vi "SetFrontPanelTypeRingFromPluginINIFile.vi"(7 "Type Key":string="Type", 8 "ErrorArray In":errorcluster[](array[cluster]), 10 "INIFilePath":path, 11 "TypeRef In":refnum<vi>) -> (0 "ErrorArray Out":errorcluster[](array[cluster]), 3 "TypeRef Out":refnum<vi>)   [LabVIEW 2017, in "Framework.lvlib"]
uses:
  Framework.lvlib
  <vilib>/Utility/config.llb/Read Key (String).vi
  <vilib>/Utility/config.llb/NI_LVConfig.lvlib
  <userlib>/NIST/NISTErrorLib/NISTErrorLib.lvlib
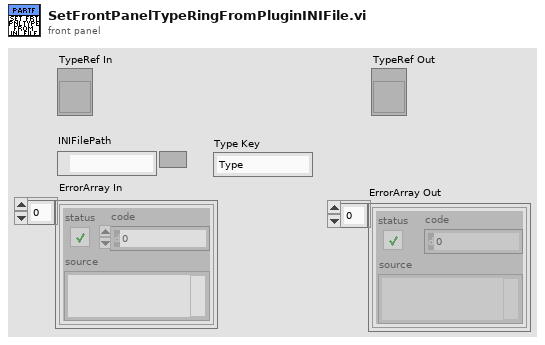
[diagram p1: front panel]
types:
  T1 = typedef "NI_LVConfig.lvlib/Config Data RefNum.ctl" = refnum<k1>
  T2 = typedef "LVStringsAndValuesArrayTypeDef_U16.ctl" = cluster{"String":string, "Value":u16}[]
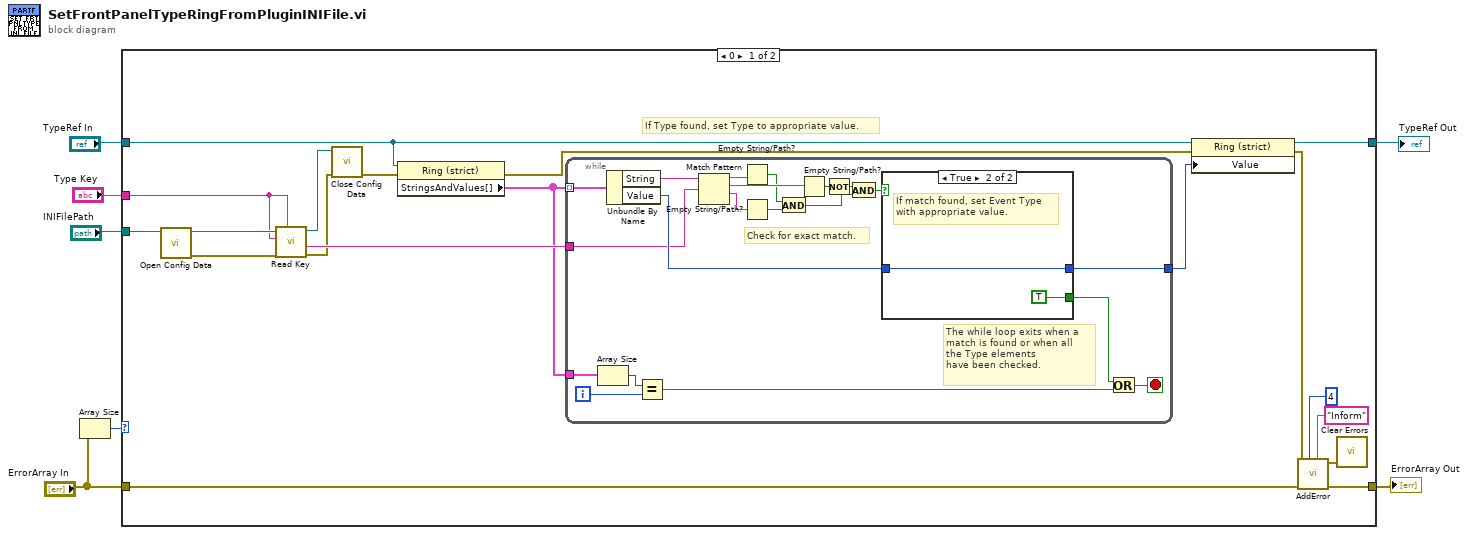
[diagram p0: block diagram]
diagram:
  n1 = Array Size(array="ErrorArray In") -> (size(s)=w6:i32)
  n2 = case shown="0" w6 {
    tunnel: [w21 w50] -> w7
    tunnel: "ErrorArray In" -> [w20 w50]
    tunnel: "INIFilePath" -> [w19 _]
    tunnel: "Type Key" -> [w11 _]
    tunnel: "TypeRef In" -> [w10 w49]
    tunnel: [w9 w49] -> w1
    frame 0 {
      # "If Type found, set Type to appropriate value."
      n3 = call <vilib>:"Open Config Data.vi"("configuration file path"=w19) -> ("error out"=w17:errorcluster, "refnum"=w18:T1)  [unwired: 8 in, 1 out]
      n4 = call-poly <vilib>:"Read Key.vi"("section"=w11, "error in (no error)"=w17, "key"=w11, "refnum"=w18) -> ("error out"=w25:errorcluster, "value"=w26:string, "refnum out"=w24:T1)  [unwired: 4 in, 1 out]
      n5 = call <vilib>:"Close Config Data.vi"("error in (no error)"=w25, "refnum"=w24) -> ("error out"=w23:errorcluster)  [unwired: 8 in, 1 out]
      n6 = property class="Ring (strict)"(reference=w10, error in=w23) -> (error out=w14:errorcluster, "StringsAndValues[]"=w22:T2)  [unwired: 1 out]
      n7 = while {
        tunnel: w22 -> [w46] mode=indexing
        tunnel: w26 -> [w35]
        tunnel: w22 -> [w30]
        tunnel: [w27] -> w13
        i -> [w31]
        stop <- w29 stop-if-true
        # "The while loop exits when a \nmatch is found or when all \nthe Type elements \nhave been checked."
        # "Check for exact match."
        n8 = Array Size(array=w30) -> (size(s)=w33:i32)
        n9 = Unbundle By Name(w46) -> ("String"=w45:string, "Value"=w43:u16)
        n10 = Equal?(x=w33, y=w31) -> (x = y?=w32:bool)
        n11 = Match Pattern(string=w45, regular expression=w35) -> (before substring=w40:string, match substring=w44:string, after substring=w39:string)  [unwired: 1 in, 1 out]
        n12 = Empty String/Path?(string/path=w40) -> (empty?=w37:bool)
        n13 = Empty String/Path?(string/path=w39) -> (empty?=w38:bool)
        n14 = And(x=w37, y=w38) -> (x .and. y?=w36:bool)
        n15 = Empty String/Path?(string/path=w44) -> (empty?=w41:bool)
        n16 = Not(x=w41) -> (.not. x?=w34:bool)
        n17 = And(x=w34, y=w36) -> (x .and. y?=w42:bool)
        n18 = case shown="True" w42 {
          tunnel: w43 -> [_ w47]
          tunnel: [_ TRUE] -> w28
          tunnel: [_ w47] -> w27
          frame False {
            # "If event type not found, set\nvalue to first index in Event\nType element list."
          }
          frame True {
            # "If match found, set Event Type\nwith appropriate value."
          }
        }
        n19 = Or(x=w28, y=w32) -> (x .or. y?=w29:bool)
      }
      n20 = property class="Ring (strict)"(reference=w10, error in=w14, "Value"=w13) -> (reference out=w9:refnum<vi>, error out=w12:errorcluster)
      n21 = call <userlib>:"AddError.vi"("Severity"="Inform" ("String"), "Priority"=u8 4, "ErrorArray"=w20, "error in (no error)"=w12) -> ("ErrorArray"=w21:errorcluster[], "error out"=w8:errorcluster)  [unwired: 6 in]
      n22 = call <vilib>:"Clear Errors.vi"("error in (no error)"=w8) -> ()  [unwired: 5 in, 2 out]
    }
    frame 1, Default {
    }
  }
  "ErrorArray Out" <- w7
  "TypeRef Out" <- w1
